vi "DCMotorCtrl_example.vi"() -> ()   [LabVIEW 2019]
uses:
  <vilib>/Rock Robotics/WPI/ThirdParty/JAS_Junk/TrajLib/TypeDef/DCMOTOR_SIM.ctl
  <vilib>/Rock Robotics/WPI/ThirdParty/JAS_Junk/TrajLib/TypeDef/LINEAR_SYSTEM_SIM.ctl
  <vilib>/Rock Robotics/WPI/ThirdParty/JAS_Junk/TrajLib/TypeDef/LINEAR_SYSTEM.ctl
  <vilib>/Analysis/Matrix/Datatypes/RealMatrix.ctl
  <vilib>/Rock Robotics/WPI/ThirdParty/JAS_Junk/TrajLib/TypeDef/DCMOTOR.CTL
  <vilib>/Rock Robotics/WPI/ThirdParty/JAS_Junk/TrajLib/Enum/DCMOTOR_TYPES_ENUM.ctl
  <vilib>/Rock Robotics/WPI/ThirdParty/JAS_Junk/TrajLib/VI/numCmd_ObtainQueue_TwoDbl.vi
  <vilib>/Rock Robotics/WPI/ThirdParty/JAS_Junk/TrajLib/VI/numCmd_ObtainQueue_OneDbl.vi
  <vilib>/Rock Robotics/WPI/ThirdParty/JAS_Junk/TrajLib/BatterySim_CalculateLoadedBatteryVoltage.vi
  <vilib>/Rock Robotics/WPI/ThirdParty/JAS_Junk/TrajLib/Trajectory_Library.lvlib
  <vilib>/Analysis/Matrix/NI_Matrix.lvlib
panel:
  in  "Tab Control":enum32{"Control", "Simulation"}(tab)
  in  "Motor Dmd - SP\n( RPM )":dbl(slide) scale=-5500.0..5500.0
  out "Motor Speed - PV (RPM)":dbl format="%20.3f"
  out "Battery Voltage (Volts)":dbl format="%20.3f"
  out "Voltage, Current Chart":cluster{dbl, "Voltage":dbl}(graph)
  out "PV, SP,CO Chart":T1(graph)
  out "Motor Current (Amps)":dbl format="%20.3f"
  out "Motor Position (Rotations)":dbl format="%20.3f"
  out "DcMotorSim":T2 {"GearBox"."Jr_KgM2" format="%13.5p"; "GearBox"."L_H" format="%13.5p"; "GearBox"."Kt_NMPerAmp" format="%13.5p"; "GearBox"."KvINV_RadPerSecPerVolt" format="%13.5p"; "GearBox"."R_Ohms" format="%13.5p"; "GearBox"."FreeSpeed_RadPerSec" format="%13.5p"; "GearBox"."FreeCurrent_Amps" format="%13.5p"; "GearBox"."StallCurrent_Amps" format="%13.5p"; "GearBox"."StallTorque_NM" format="%13.5p"; "GearBox"."nominalVoltage_Volts" format="%13.5p"}
  # "<States, 1>"
  # "<Outputs, 1>"
  # "<Inputs, 1>"
  # "<Outputs, 1>"
  # "<States,States>"
  # "<States,Inputs>"
  # "<Outputs,States>"
  # "<Outputs,Inputs>"
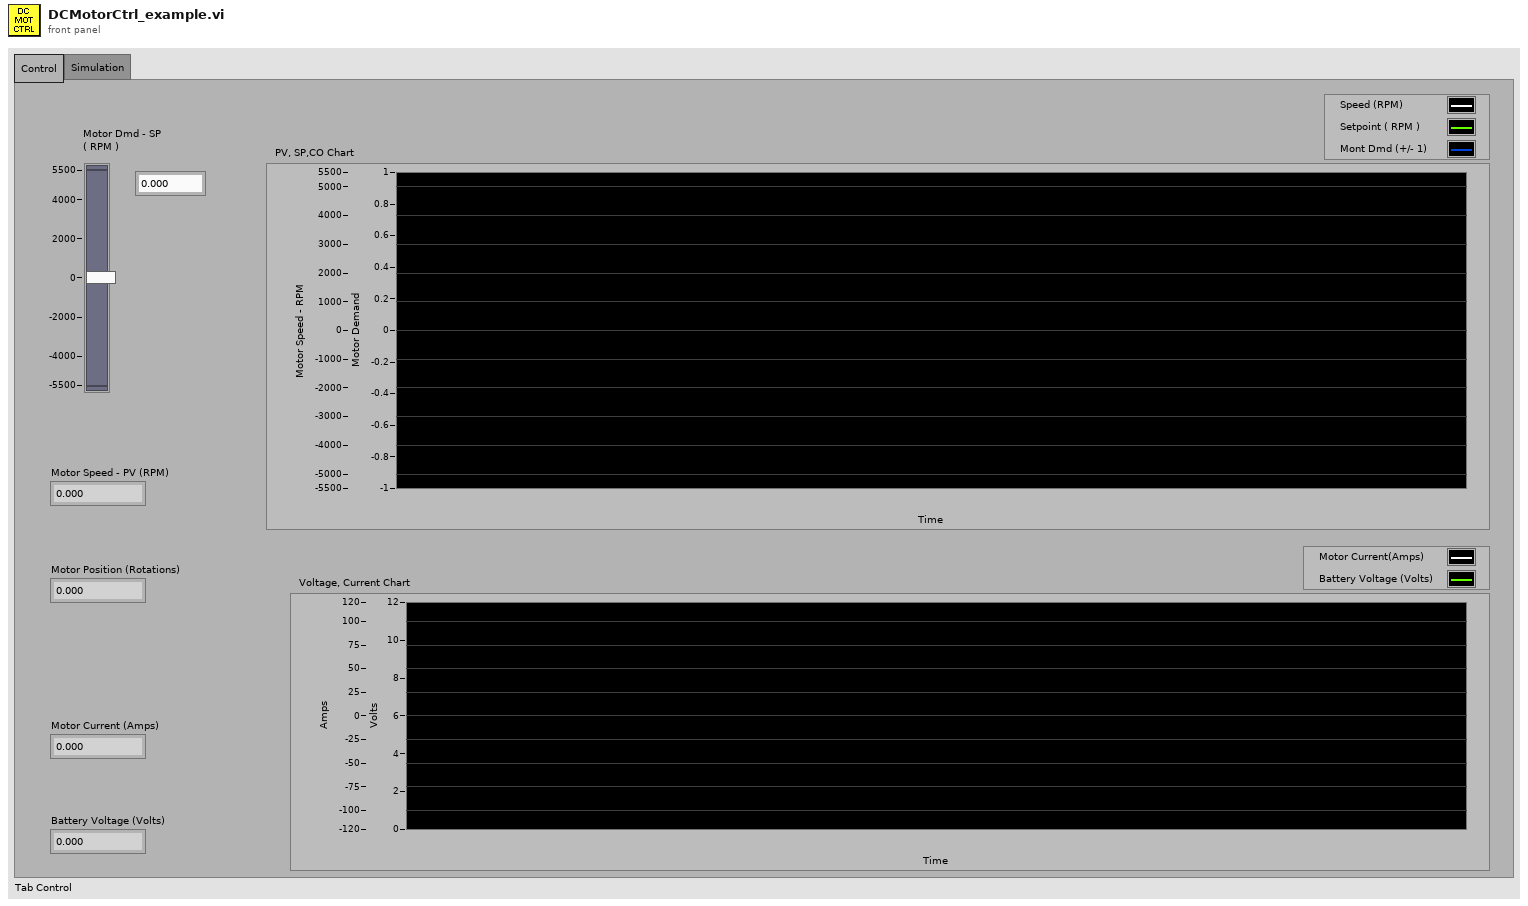
[diagram p1: front panel]
types:
  T1 = cluster{"Velocity_RPM":dbl, "Value":dbl, "Value":dbl}
  T2 = typedef "Trajectory_Library.lvlib/DCMOTOR_SIM.ctl" = cluster{"LinearSystemSim":T3, "GearBox":T6, "Gearing":dbl}
  T3 = typedef "Trajectory_Library.lvlib/LINEAR_SYSTEM_SIM.ctl" = cluster{"m_Plant":T4, "m_X":T5, "m_Y":T5, "m_U":T5, "MeasureStdDev":T5}
  T4 = typedef "Trajectory_Library.lvlib/LINEAR_SYSTEM.ctl" = cluster{"m_A":T5, "m_B":T5, "m_C":T5, "m_D":T5, "States":i32, "Inputs":i32, "Outputs":i32}
  T5 = typedef "NI_Matrix.lvlib/RealMatrix.ctl" = dbl[][]
  T6 = typedef "Trajectory_Library.lvlib/DCMOTOR.CTL" = cluster{"nominalVoltage_Volts":dbl, "StallTorque_NM":dbl, "StallCurrent_Amps":dbl, "FreeCurrent_Amps":dbl, "FreeSpeed_RadPerSec":dbl, "R_Ohms":dbl, "KvINV_RadPerSecPerVolt":dbl, "Kt_NMPerAmp":dbl, "L_H":dbl, "Jr_KgM2":dbl}
  T7 = typedef "Trajectory_Library.lvlib/DCMOTOR_TYPES_ENUM.ctl" = enum16{"CIM", "AndyMark 9015", "Andy Mark RS 775 125", "Bag", "BaneBots RS 550", "BaneBots RS 775", "Falcon 500", "Mini CIM", "NEO", "NEO 550", "Romi BuiltIn", "Vex 775 Pro", "Snow Blower AM 2235A", "Bosch Seat AM 3493"}
  T8 = typedef "Trajectory_Library.lvlib/LINEAR_SYSTEM_ID_DCMOTOR_MODEL.ctl" = cluster{"DCMOTOR_TYPES":T7, "Num Motors":i32, "Gearing":dbl, "MOI kgm2":dbl}
  T9 = typedef "Trajectory_Library.lvlib/DCMOTOR_SIM_SIMULATION_PARAMS.ctl" = cluster{"Pos Sim Std Dev Rotations":dbl, "Vel Sim Std Dev RPM":dbl}
  T10 = typedef "Trajectory_Library.lvlib/LINEAR_SYSTEM_LOOP_DCMOTOR_CTRL_PARAMS.ctl" = cluster{"Vel Model Std Dev Rad/Sec":dbl, "Vel Meas Std Dev Rad/Sec":dbl, "Vel Ctrl Tol Rad/Sec":dbl, "Max Ctrl Out V":dbl, "Pos Model Std Dev Rad":dbl, "Pos Meas Std Dev Rad":dbl, "Pos Ctrl Tol Rad":dbl}
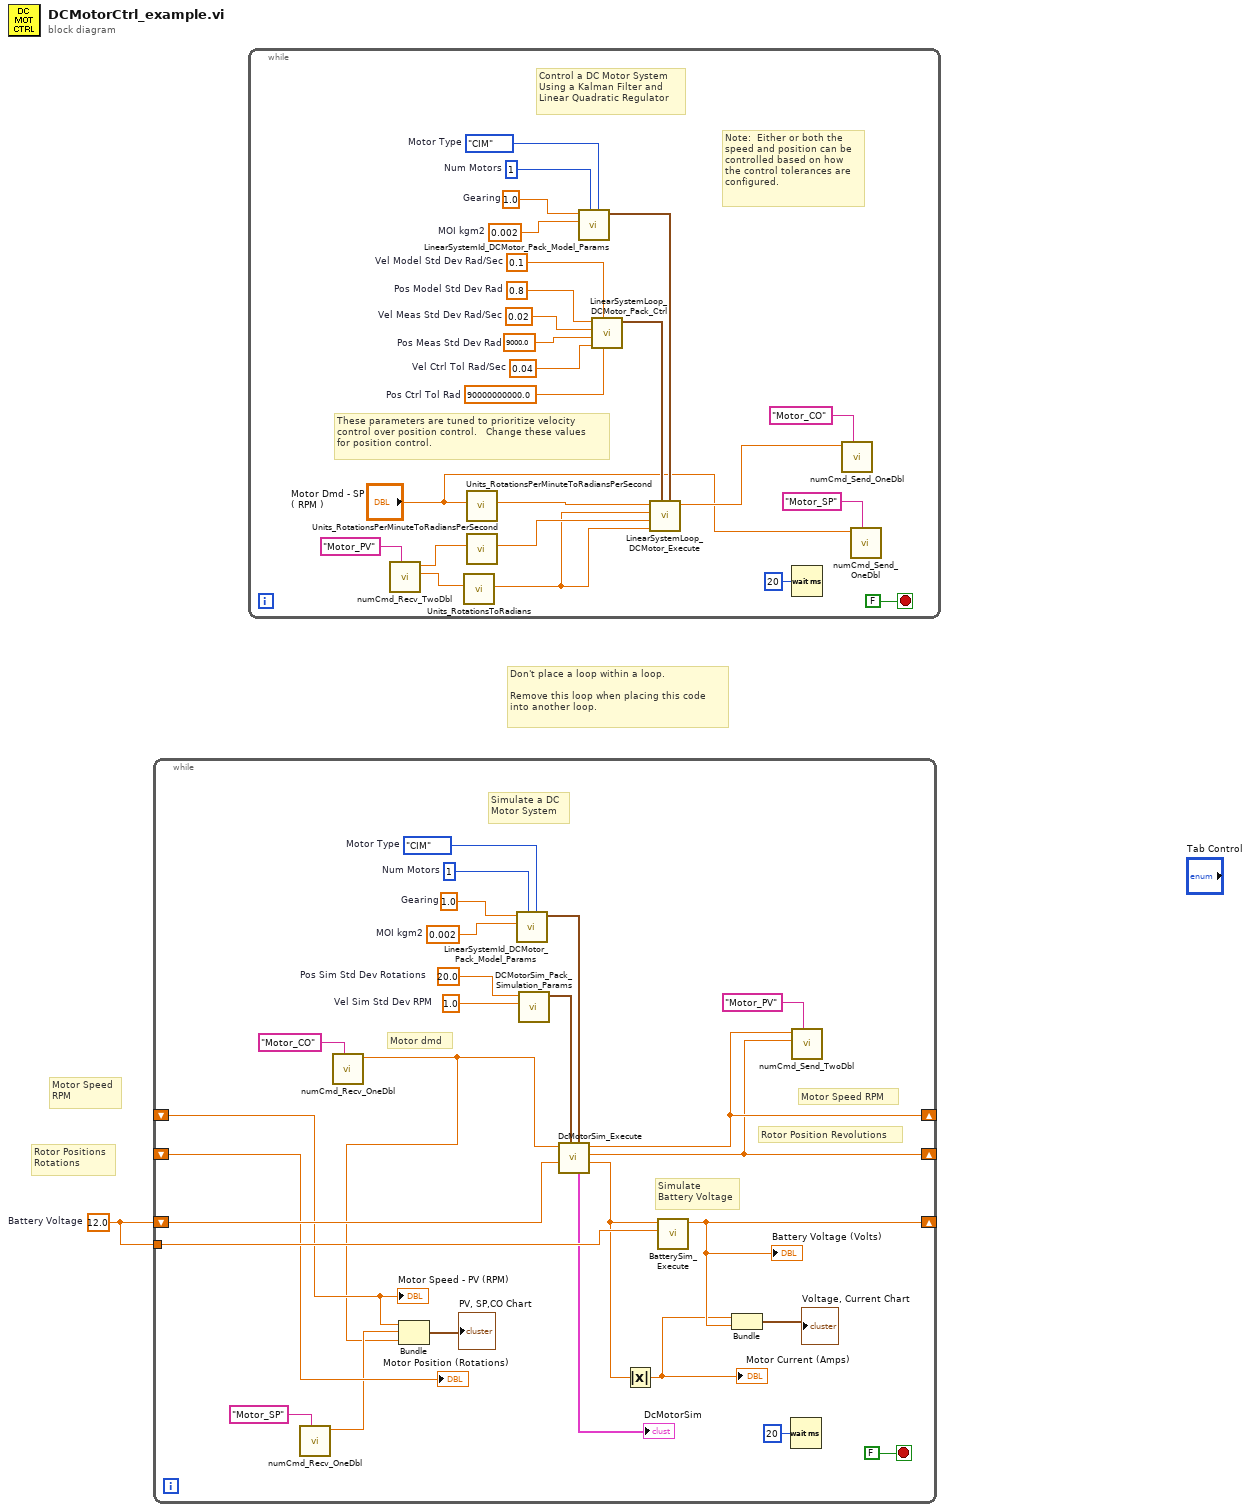
[diagram p0: block diagram]
diagram:
  w1 = 12.0  # Battery Voltage
  # "Don't place a loop within a loop.\n \nRemove this loop when placing this code\ninto another loop."
  # "Rotor Positions\nRotations"
  # "Motor Speed\nRPM"
  n1 = while {
    shift-right: [w11] -> _
    shift-left: w1 -> [w22]
    shift-right: [w7] -> _
    shift-left: _ -> [w15]
    shift-right: [w6] -> _
    shift-left: _ -> [w14]
    tunnel: w1 -> [w17]
    stop <- FALSE stop-if-true
    w18 = 20.0  # Pos Sim Std Dev Rotations
    w19 = 1.0  # Vel Sim Std Dev RPM
    w25 = 1.0  # Gearing
    w26 = 0.002  # MOI kgm2
    w27 = 1  # Num Motors
    w28 = DCMOTOR_TYPES_ENUM."CIM"  # Motor Type
    # "Motor dmd"
    # "Rotor Position Revolutions"
    # "Motor Speed RPM"
    # "Simulate\nBattery Voltage"
    # "Simulate a DC \nMotor System"
    n2 = call <vilib>:"numCmd_Recv_OneDbl.vi"("Command Name"="Motor_SP") -> ("Value"=w3:dbl)  [unwired: 8 in, 2 out]
    n3 = call <vilib>:"numCmd_Recv_OneDbl.vi"("Command Name"="Motor_CO") -> ("Value"=w2:dbl)  [unwired: 8 in, 2 out]
    n4 = Bundle("Velocity_RPM"=w15, "Value"=w3, "Value"=w2) -> (→"PV, SP,CO Chart":T1)  [unwired: 1 in]
    n5 = call <vilib>:"LinearSystemId_DCMotor_Pack_Model_Params.vi"("DCMOTOR_TYPES"=w28, "Num Motors"=w27, "MOI kgm2"=w26, "Gearing"=w25) -> ("LinearSystem_ID_DCMotor_Model"=w21:T8)  [unwired: 7 in]
    n6 = call <vilib>:"DCMotorSim_Pack_Simulation_Params.vi"("Vel Sim Std Dev RPM"=w19, "Pos Sim Std Dev Rotations"=w18) -> ("DCMOTOR_Sim_Simulation_Params"=w20:T9)  [unwired: 9 in]
    n7 = call <vilib>:"DcMotorSim_Execute.vi"("DCMotor_Model _Params"=w21, "DCMOTORSim_Simulation_Params"=w20, "Battery Voltage"=w22, "Motor Dmd (CO)"=w2) -> ("Motor Current"=w13:dbl, "Position_Rotations"=w6:dbl, "Velocity_RPM"=w7:dbl, "out DcMotorSim"=→"DcMotorSim":T2)  [unwired: 3 in, 1 out]
    n8 = Absolute Value(x=w13) -> (abs(x)=w10:dbl)
    "Motor Current (Amps)" <- w10
    n9 = call <vilib>:"BatterySim_Execute.vi"("Nominal Battery Voltage"=w17, "Current"=w13) -> ("Voltage"=w11:dbl)  [unwired: 9 in]
    "Battery Voltage (Volts)" <- w11
    n10 = Bundle(w10, "Voltage"=w11) -> (→"Voltage, Current Chart":cluster{dbl, "Voltage":dbl})  [unwired: 1 in]
    n11 = Wait (ms)(milliseconds to wait=u32 20) -> ()  [unwired: 1 out]
    n12 = call <vilib>:"numCmd_Send_TwoDbl.vi"("Command Name"="Motor_PV", "Value 2"=w6, "Value 1"=w7) -> ()  [unwired: 8 in, 1 out]
    "Motor Speed - PV (RPM)" <- w15
    "Motor Position (Rotations)" <- w14
  }
  n13 = while {
    stop <- FALSE stop-if-true
    w39 = 0.8  # Pos Model Std Dev Rad
    w40 = 0.02  # Vel Meas Std Dev Rad/Sec
    w41 = 9000.0  # Pos Meas Std Dev Rad
    w42 = 0.04  # Vel Ctrl Tol Rad/Sec
    w43 = 0.1  # Vel Model Std Dev Rad/Sec
    w44 = 90000000000.0  # Pos Ctrl Tol Rad
    w49 = 1.0  # Gearing
    w50 = 0.002  # MOI kgm2
    w51 = 1  # Num Motors
    w52 = DCMOTOR_TYPES_ENUM."CIM"  # Motor Type
    # "These parameters are tuned to prioritize velocity\ncontrol over position control.   Change these values\nfor position control."
    # "Note:  Either or both the\nspeed and position can be\ncontrolled based on how\nthe control tolerances are\nconfigured."
    # "Control a DC Motor System\nUsing a Kalman Filter and \nLinear Quadratic Regulator"
    n14 = call <vilib>:"numCmd_Recv_TwoDbl.vi"("Command Name"="Motor_PV") -> ("Value 2"=w35:dbl, "Value 1"=w36:dbl)  [unwired: 7 in, 2 out]
    n15 = call <vilib>:"Units_RotationsToRadians.vi"("Rotations"=w35) -> ("Radians"=w33:dbl)  [unwired: 10 in]
    n16 = call <vilib>:"Units_RotationsPerMinuteToRadiansPerSecond.vi"("RotationsPerMinute"="Motor Dmd - SP\n( RPM )") -> ("RadiansPerSecond"=w38:dbl)  [unwired: 10 in]
    n17 = call <vilib>:"Units_RotationsPerMinuteToRadiansPerSecond.vi"("RotationsPerMinute"=w36) -> ("RadiansPerSecond"=w34:dbl)  [unwired: 10 in]
    n18 = call <vilib>:"LinearSystemId_DCMotor_Pack_Model_Params.vi"("DCMOTOR_TYPES"=w52, "Num Motors"=w51, "MOI kgm2"=w50, "Gearing"=w49) -> ("LinearSystem_ID_DCMotor_Model"=w46:T8)  [unwired: 7 in]
    n19 = call <vilib>:"LinearSystemLoop_DCMotor_Pack_Ctrl.vi"("Pos Ctrl Tol Rad"=w44, "Vel Model Std Dev Rad/Sec"=w43, "Vel Ctrl Tol Rad/Sec"=w42, "Pos Meas Std Dev Rad"=w41, "Vel Meas Std Dev Rad/Sec"=w40, "Pos Model Std Dev Rad"=w39) -> ("LinearSystemLoop_DCMotor_Ctrl_Params"=w45:T10)  [unwired: 5 in]
    n20 = call <vilib>:"LinearSystemLoop_DCMotor_Execute.vi"("LinearSystem_ID_DCMotor_Model"=w46, "LinearSystem_DCMotor_Ctrl_Params"=w45, "Position PV (Rad)"=w33, "Velocity (Rad/Sec)\n(PV)"=w34, "Position SP (Rad)"=w33, "Velocity (Rad/Sec)\nSetpoint (SP)"=w38) -> ("Motor Dmd"=w32:dbl)  [unwired: 1 in, 4 out]
    n21 = Wait (ms)(milliseconds to wait=u32 20) -> ()  [unwired: 1 out]
    n22 = call <vilib>:"numCmd_Send_OneDbl.vi"("Command Name"="Motor_CO", "Value"=w32) -> ()  [unwired: 9 in, 1 out]
    n23 = call <vilib>:"numCmd_Send_OneDbl.vi"("Command Name"="Motor_SP", "Value"="Motor Dmd - SP\n( RPM )") -> ()  [unwired: 9 in, 1 out]
  }
